vi "12.1-BasicMophology.vi"() -> ()   [LabVIEW 2016]
doc: "This example shows how to use the Edge Tool in NI Vision. The Edge Tool finds edges (or sharp transitions in the pixels values) along a given line or ROI profile. The Edge Tool is a precursor function to many of the gauging and inspection tasks. For example, the location of the edges found along a line profile across an object can interpreted as the boundaries of the object whose dimensions have to be measured for a gauging application or the presence of a crack in the surface of an object for an inspection application."
uses:
  <vilib>/vision/NI_Vision_Development_Module.lvlib
panel:
  out "Src":T1(plugin-control)
  in  "Structuring Element":i32[][](array[numeric])=[[0, 1, 0], [1, 1, 1], [0, 0, 0]]
  in  "Hexa Pixel?":bool
  in  "# of iterations":i32=1
  in  "Operation":u16(ring) items=["AutoM", "Close", "Dilate", "Erode", "Gradient", "Gradient out", "Gradient in", "Hit miss", "Open", "PClose", "POpen", "Thick", "Thin"]
  out "Dst":T1(plugin-control)
  in  "Stop":bool
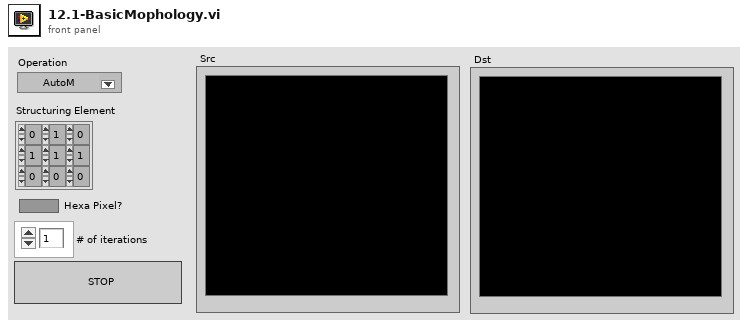
[diagram p1: front panel]
types:
  T1 = typedef "IMAQ Image.ctl" = refnum<image>
  T2 = cluster{"Hexa Pixel?":bool, "Operation":u16, "Structuring Element":i32[][], "# of iterations":i32}
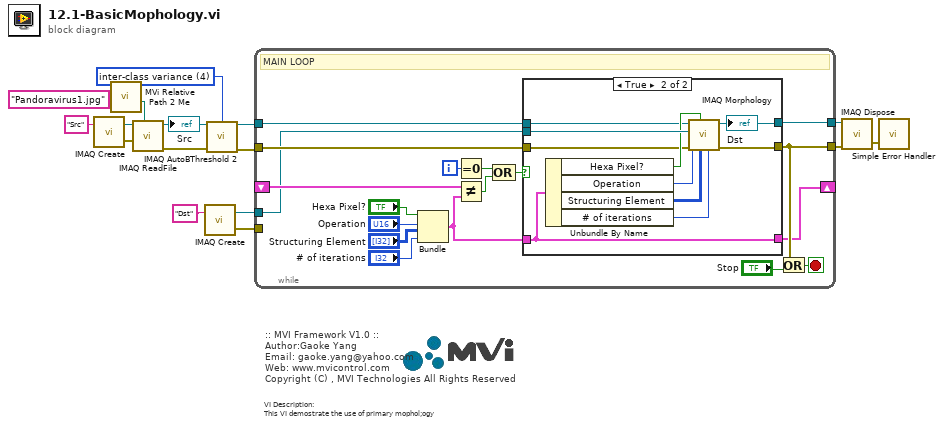
[diagram p0: block diagram]
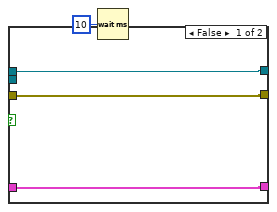
[diagram p2: hidden frame]
diagram:
  w5 = 4 items=["clustering", "entropy", "metric", "moments", "inter-class variance"] ("Method")
  # "VI Description:\nThis VI demostrate the use of primary mophol;ogy"
  # ":: MVI Framework V1.0 ::\nAuthor:Gaoke Yang\nEmail: gaoke.yang@yahoo.com\nWeb: www.mvicontrol.com\nCopyright (C) , MVI Technologies All Rights Reserved"
  n1 = call "IMAQ Create"("Image Name"="Src") -> ("New Image"=w15:T1, "error out"=w14:errorcluster)  [unwired: 4 in]
  n2 = call "MVi Relative Path 2 Me.vi"("Relative Path"="Pandoravirus1.jpg" ("name or relative path")) -> ("Appended Dir"=w10:path)  [unwired: 5 in, 1 out]
  n3 = call "IMAQ ReadFile"("File Path"=w10, "error in (no error)"=w14, "Image"=w15) -> ("error out"=w2:errorcluster, "Image Out"=w1:T1)  [unwired: 4 in, 3 out]
  "Src" <- w1
  n4 = call "IMAQ Create"("Image Name"="Dst") -> ("New Image"=w7:T1, "error out"=w6:errorcluster)  [unwired: 4 in]
  n5 = call "IMAQ AutoBThreshold 2"("Image Src"=w1, "Method (clustering)"=w5, "error in (no error)"=w2) -> ("Image Dst Out"=w3:T1, "error out"=w4:errorcluster)  [unwired: 5 in, 6 out]
  n6 = while "MAIN LOOP" {
    tunnel: w3 -> [w33]
    tunnel: w4 -> [w34]
    tunnel: [w29] -> w13
    tunnel: [w30] -> w12
    shift-right: [w26] -> _
    shift-left: _ -> [w23]
    tunnel: w7 -> [w21]
    tunnel: w6 -> [_]
    i -> [w28]
    stop <- w31 stop-if-true
    # "MAIN LOOP"
    n7 = Bundle("Hexa Pixel?"="Hexa Pixel?", "Operation"="Operation", "Structuring Element"="Structuring Element", "# of iterations"="# of iterations") -> (w24:T2)  [unwired: 1 in]
    n8 = Equal To 0?(x=w28) -> (x = 0?=w25:bool)
    n9 = Not Equal?(x=w23, y=w24) -> (x != y?=w22:bool)
    n10 = Compound Arithmetic op=OR(w25, w22) -> (w27:bool)
    n11 = case shown="True" w27 {
      tunnel: w34 -> [w37 w39]
      tunnel: w33 -> [w38 w40]
      tunnel: [w38 w41] -> w30
      tunnel: [w37 w42] -> w29
      tunnel: [w35 w47] -> w26
      tunnel: w24 -> [w35 w47]
      tunnel: w21 -> [_ w48]
      frame False {
        n12 = Wait (ms)(milliseconds to wait=u32 10) -> ()  [unwired: 1 out]
      }
      frame True {
        n13 = Unbundle By Name(w47) -> ("Hexa Pixel?"=w43:bool, "Operation"=w44:u16, "Structuring Element"=w45:i32[][], "# of iterations"=w46:i32)
        n14 = call "IMAQ Morphology"("Number of iterations (1)"=w46, "Structuring Element"=w45, "Square/Hexa (Square)"=w43, "error in (no error)"=w39, "Operation"=w44, "Image Dst"=w48, "Image Src"=w40) -> ("error out"=w42:errorcluster, "Image Dst Out"=w41:T1)  [unwired: 3 in]
        "Dst" <- w41
      }
    }
    n15 = Or(x=w29, y="Stop") -> (x .or. y?=w31:bool)
  }
  n16 = call "IMAQ Dispose"("Image"=w12, "error in (no error)"=w13) -> ("error out"=w9:errorcluster)  [unwired: 4 in]
  n17 = call <vilib>:"Simple Error Handler.vi"("error in (no error)"=w9) -> ()  [unwired: 4 in, 5 out]
